vi "Parse.vi"(8 "error in":errorcluster, 10 "Object Dictionary":refnum<class "Dictionary.lvclass">, 11 "Info Section in":refnum<class "Info Section.lvclass">) -> (0 "error out":errorcluster, 3 "Info Section out":refnum<class "Info Section.lvclass">)   [LabVIEW 2024, in "Electronic Datasheet.lvlib" / "Info Section.lvclass"]
uses:
  Info Section.lvclass
  Object Dictionary/Dictionary.lvclass
  Info Section.lvclass/Info Section.ctl
  <vilib>/Utility/Data Type/NI_Data Type.lvlib
  OD Section/Section.lvclass
  <userlib>/_OpenG.lib/lvdata/lvdata.llb/openg_variant.lvlib
  Value/Value.lvclass
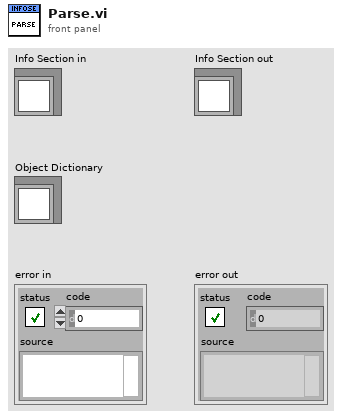
[diagram p1: front panel]
types:
  T1 = typedef "NI_Data Type.lvlib/Data Type.ctl" = enum8{"Invalid Type", "Void", "I8", "I16", "I32", "I64", "U8", "U16", "U32", "U64", "Single Float", "Double Float", "Extended Float", "Single Complex", "Double Complex", "Extended Complex", "Enum U8", "Enum U16", "Enum U32", "Enum U64", "Single Float With Unit", "Double Float With Unit", "Extended Float With Unit", "Single Complex with Unit", "Double Complex with Unit", "Extended Complex with Unit", "Boolean", "String", "Path", "Picture", "Tag", "Array", "Cluster", "Variant", "LV Variant", "Waveform", "Timestamp", "Digital Waveform", "Digital Data", "ExpressData", "Refnum", "External Data", "VI", "Poly VI", "LabVIEW Class Instance", "Fixed Point", "Set Collection", "Map Collection"}
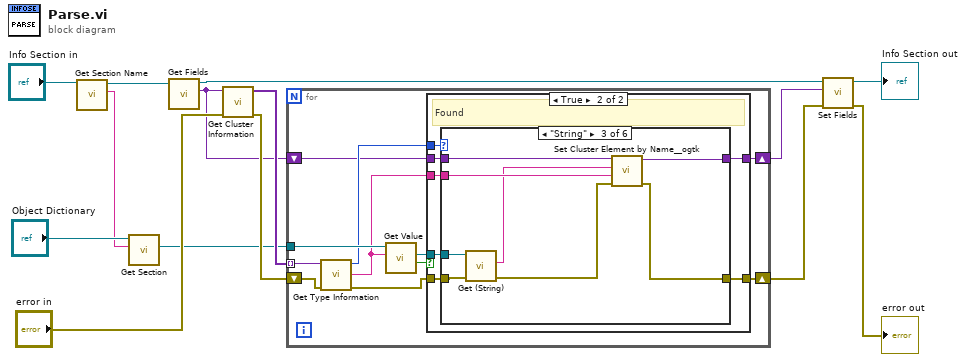
[diagram p0: block diagram]
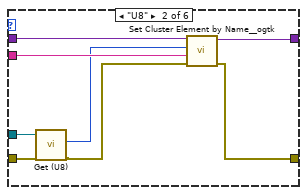
[diagram p4: hidden frame]
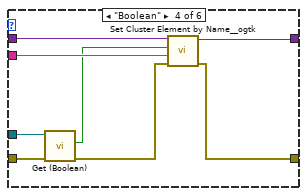
[diagram p5: hidden frame]
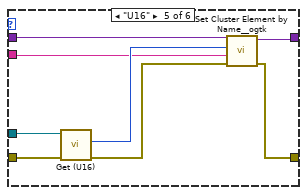
[diagram p6: hidden frame]
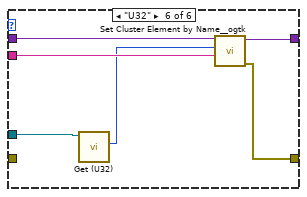
[diagram p7: hidden frame]
diagram:
  n1 = call-dynamic "Get Section Name.vi"("Info Section in"="Info Section in") -> ("Section"=w11:string, "Info Section out"=w12:refnum<class "Info Section.lvclass">)  [unwired: 9 in]
  n2 = call "Get Section.vi"("Section"=w11, "Dictionary in"="Object Dictionary") -> ("Section out"=w7:refnum<class "Section.lvclass">)  [unwired: 7 in, 2 out]
  n3 = call-dynamic "Get Fields.vi"("Info Section in"=w12) -> ("Fields Cluster"=w2:variant, "Info Section out"=w6:refnum<class "Info Section.lvclass">)  [unwired: 9 in]
  n4 = call <vilib>:"Get Cluster Information.vi"("error in (no error)"="error in", "variant"=w2) -> ("error out"=w8:errorcluster, "cluster elements"=w9:variant[])  [unwired: 8 in]
  n5 = for {
    tunnel: w9 -> [w25] mode=indexing
    tunnel: w7 -> [w23]
    shift-right: [w17] -> w4
    shift-left: w8 -> [w24]
    shift-right: [w18] -> w1
    shift-left: w2 -> [w20]
    n6 = call <vilib>:"Get Type Information.vi"("error in (no error)"=w24, "variant"=w25) -> ("error out"=w15:errorcluster, "name"=w19:string, "type"=w22:T1)  [unwired: 5 in, 2 out]
    n7 = call "Get Value.vi"("Key"=w19, "Object Entry in"=w23) -> ("Found?"=w16:bool, "Value"=w21:refnum<class "Value.lvclass">)  [unwired: 7 in, 1 out]
    n8 = case shown="True" w16 {
      tunnel: w15 -> [w27 w34]
      tunnel: w22 -> [_ w33]
      tunnel: w21 -> [_ w32]
      tunnel: w20 -> [w26 w28]
      tunnel: w19 -> [_ w31]
      tunnel: [w26 w30] -> w18
      tunnel: [w27 w29] -> w17
      frame False {
        # "Not found"
      }
      frame True {
        # "Found"
        n9 = case shown="\"String\"" w33 {
          tunnel: w34 -> [w35 w40 w45 w53 w60 _]
          tunnel: w31 -> [_ w42 w48 w56 w64 w73]
          tunnel: [w35 w43 w51 w55 w61 w70] -> w29
          tunnel: [w36 w41 w50 w58 w62 w71] -> w30
          tunnel: w32 -> [_ w39 w47 w59 w63 w69]
          tunnel: w28 -> [w36 w44 w49 w57 w65 w72]
          frame "Invalid Type", Default {
          }
          frame "U8" {
            n10 = call "Get (U8).vi"("error in"=w40, "Value in"=w39) -> ("error out"=w38:errorcluster, "Value"=w37:u8)  [unwired: 6 in, 2 out]
            n11 = call <userlib>:"Set Cluster Element by Name__ogtk.vi"("error in (no error)"=w38, "Element Name (\"\": New Element Data Name)"=w42, "New Element Value"=w37, "Cluster"=w44) -> ("error out"=w43:errorcluster, "VCluster out"=w41:variant)  [unwired: 5 in, 1 out]
          }
          frame "String" {
            n12 = call "Get (String).vi"("Value in"=w47) -> ("Value"=w46:string)  [unwired: 8 in, 2 out]
            n13 = call <userlib>:"Set Cluster Element by Name__ogtk.vi"("error in (no error)"=w45, "Element Name (\"\": New Element Data Name)"=w48, "New Element Value"=w46, "Cluster"=w49) -> ("error out"=w51:errorcluster, "VCluster out"=w50:variant)  [unwired: 5 in, 1 out]
          }
          frame "Boolean" {
            n14 = call "Get (Boolean).vi"("error in"=w53, "Value in"=w59) -> ("error out"=w52:errorcluster, "Value"=w54:bool)  [unwired: 6 in, 2 out]
            n15 = call <userlib>:"Set Cluster Element by Name__ogtk.vi"("error in (no error)"=w52, "Element Name (\"\": New Element Data Name)"=w56, "New Element Value"=w54, "Cluster"=w57) -> ("error out"=w55:errorcluster, "VCluster out"=w58:variant)  [unwired: 5 in, 1 out]
          }
          frame "U16" {
            n16 = call "Get (U16).vi"("error in"=w60, "Value in"=w63) -> ("error out"=w66:errorcluster, "Value"=w67:u16)  [unwired: 6 in, 2 out]
            n17 = call <userlib>:"Set Cluster Element by Name__ogtk.vi"("error in (no error)"=w66, "Element Name (\"\": New Element Data Name)"=w64, "New Element Value"=w67, "Cluster"=w65) -> ("error out"=w61:errorcluster, "VCluster out"=w62:variant)  [unwired: 5 in, 1 out]
          }
          frame "U32" {
            n18 = call "Get (U32).vi"("Value in"=w69) -> ("Value"=w68:u32)  [unwired: 8 in, 2 out]
            n19 = call <userlib>:"Set Cluster Element by Name__ogtk.vi"("Element Name (\"\": New Element Data Name)"=w73, "New Element Value"=w68, "Cluster"=w72) -> ("error out"=w70:errorcluster, "VCluster out"=w71:variant)  [unwired: 6 in, 1 out]
          }
        }
      }
    }
  }
  n20 = call-dynamic "Set Fields.vi"("error in"=w4, "Fields Cluster"=w1, "Info Section in"=w6) -> ("error out"=→"error out":errorcluster, "Info Section out"=→"Info Section out":refnum<class "Info Section.lvclass">)  [unwired: 7 in]
